vi "XNET Database Create (Dynamic Signal).vi"(0 "subframe in":refnum<k21>, 7 "signal name":string, 11 "error in (no error)":errorcluster) -> (4 "subframe out":refnum<k21>, 8 "signal out":refnum<k21>, 15 "error out":errorcluster)   [LabVIEW 2018]
doc: "Create a new dynamic signal (signal within a multiplexed subframe)."
uses:
  nixlvapi.dll
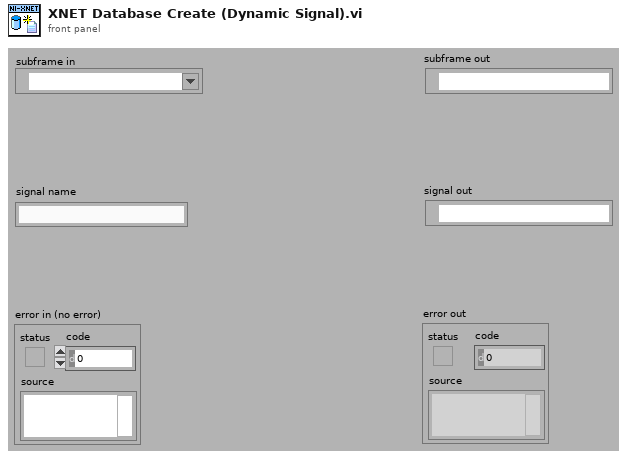
[diagram p1: front panel]
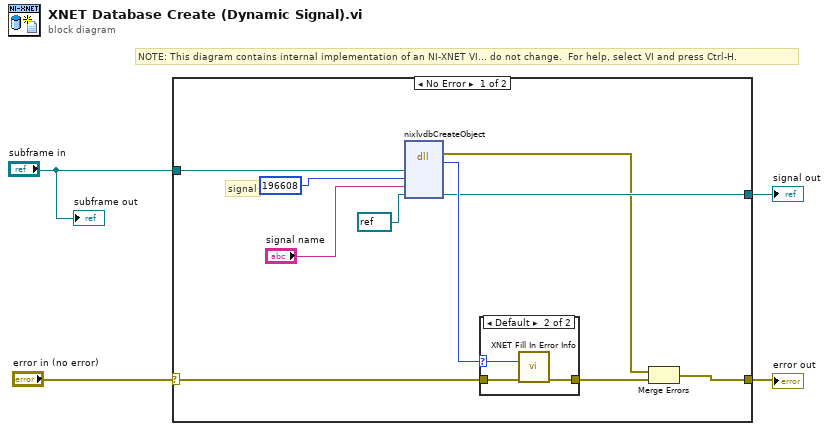
[diagram p0: block diagram]
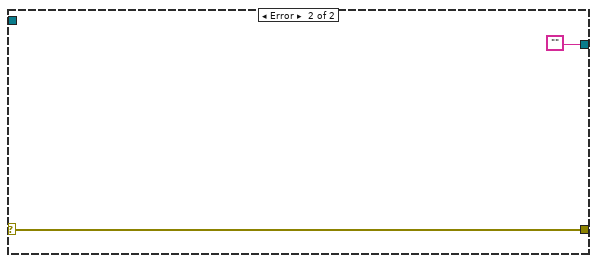
[diagram p3: hidden frame]
diagram:
  # "NOTE: This diagram contains internal implementation of an NI-XNET VI... do not change.  For help, select VI and press Ctrl-H."
  n1 = case shown="No Error" "error in (no error)" {
    selector: "error in (no error)" -> [w14 w20]
    tunnel: "subframe in" -> [w11 _]
    tunnel: [w6 w20] -> w4
    tunnel: [w7 ""] -> w1
    frame No Error {
      # "signal"
      n2 = dll-call lib="nixlvapi.*" fn="nixlvdbCreateObject" ("nilvxaiu.dll:lvxenDatabaseCreateObject")("parentObjRef"=w11, "objectClass"=u32 196608 ("class"), "objectName"="signal name", "refObjPtr"=refnum<k21> refnum ("signal out")) -> (error out=w5:errorcluster, "return type"=w13:i32, "refObjPtr"=w7:refnum<k21>)  [unwired: 5 in, 2 out]
      n3 = case shown="Default" w13 {
        selector: w13 -> [_ w16]
        tunnel: w14 -> [w15 w17]
        tunnel: [w15 w18] -> w12
        frame 0 {
        }
        frame Default {
          n4 = call "XNET Fill In Error Info.vi"("status code"=w16, "error in"=w17) -> ("error out"=w18:errorcluster)  [unwired: 13 out]
        }
      }
      n5 = Merge Errors(w5, w12) -> (w6:errorcluster)
    }
    frame Error {
    }
  }
  "error out" <- w4
  "signal out" <- w1
  "subframe out" <- "subframe in"
